vi "Pin Positions DAO.vi"(0 "LBCB Settings Actions":T4, 3 "Config Ref Number":T3, 5 "LBCB Number":T1, 7 "LBCB Pins In":T2={"Pin Positions"=[[0.0, 0.0, 0.0]], "Row Labels"=[]}, 11 "error in (no error)":errorcluster) -> (8 "LBCB Pins Output":T2, 14 "Config Ref Number out":T3, 15 "error out":errorcluster)   [LabVIEW 2013]
uses:
  Metadata/Persistant DAO Actions.ctl
  <vilib>/Utility/config.llb/Config Data RefNum.ctl
  Metadata/Pin Positions.ctl
  Metadata/LBCB Number.ctl
  <vilib>/Utility/config.llb/NI_LVConfig.lvlib
panel:
  in  "Keys":string[](array[string])=["X1", "X2", "Y1", "Z1", "Z2", "Z3"]
  # "Fixed"
  # "Platten"
  # "X"
  # "Z"
  # "X"
  # "Z"
  # "Y"
  # "Y"
  # "Fixed"
  # "Platten"
  # "X"
  # "Z"
  # "X"
  # "Z"
  # "Y"
  # "Y"
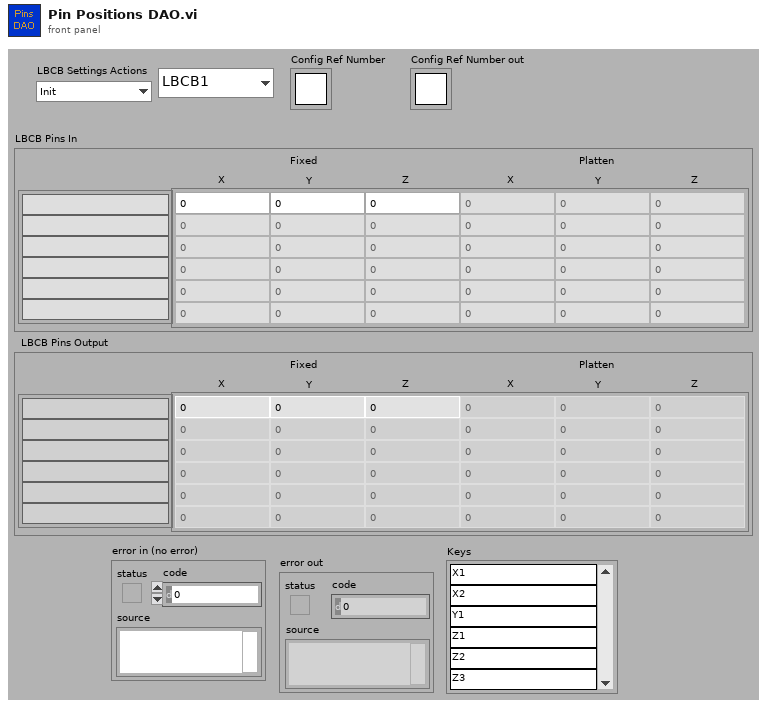
[diagram p1: front panel]
types:
  T1 = typedef "LBCB Number.ctl" = enum16{"LBCB1", "LBCB2"}
  T2 = typedef "Pin Positions.ctl" = cluster{"Pin Positions":dbl[][], "Row Labels":string[]}
  T3 = typedef "NI_LVConfig.lvlib/Config Data RefNum.ctl" = refnum<k1>
  T4 = typedef "Persistant DAO Actions.ctl" = enum16{"Init", "Get", "Set", "Load", "Save"}
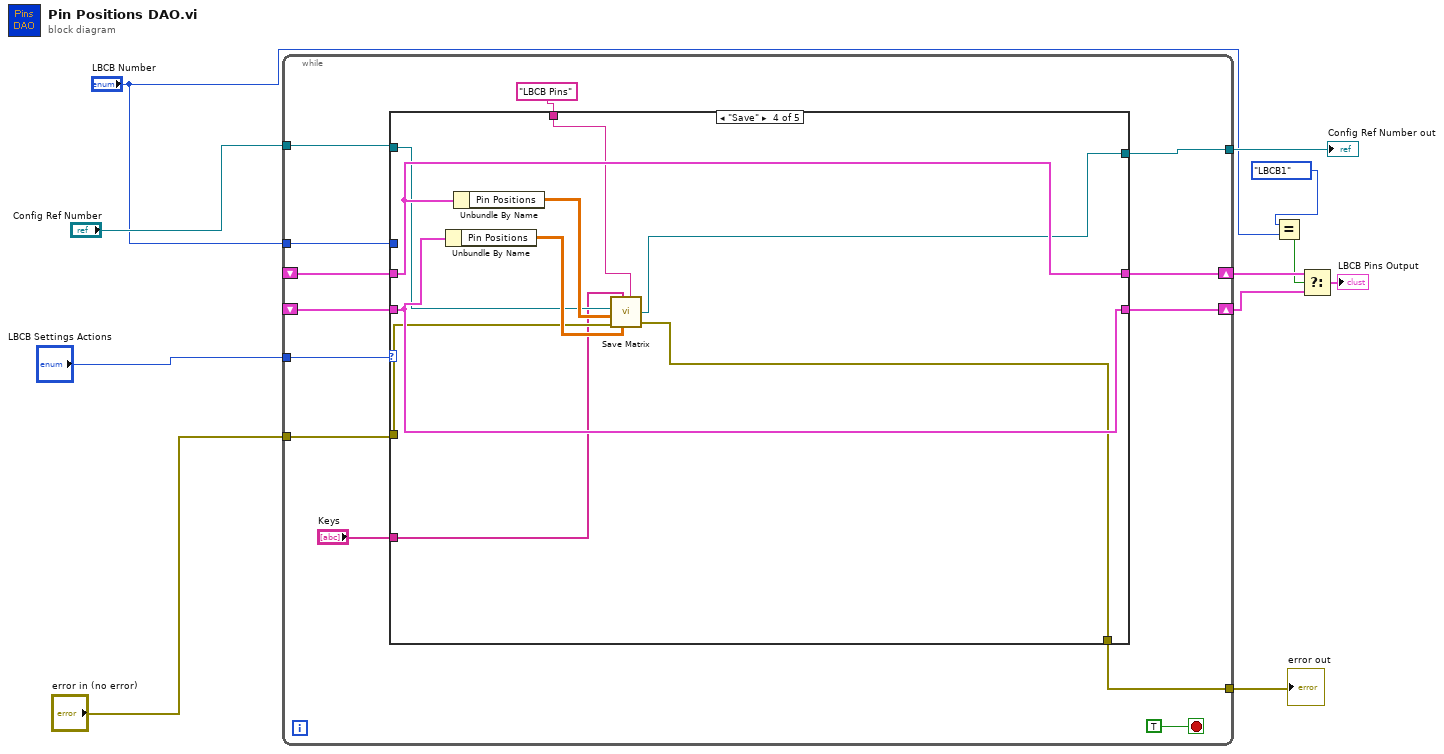
[diagram p0: block diagram]
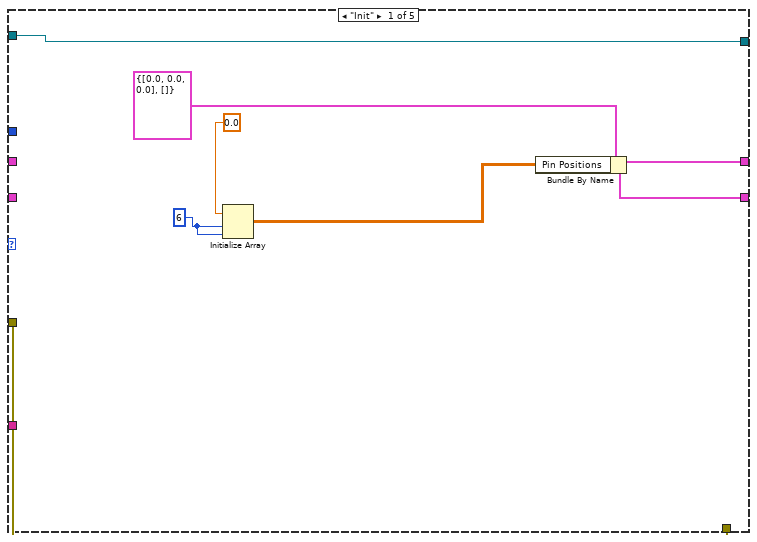
[diagram p2: hidden frame]
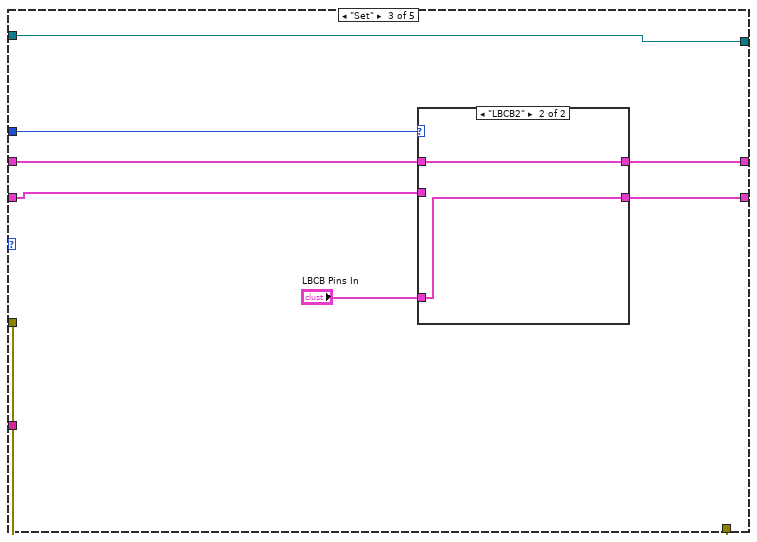
[diagram p4: hidden frame]
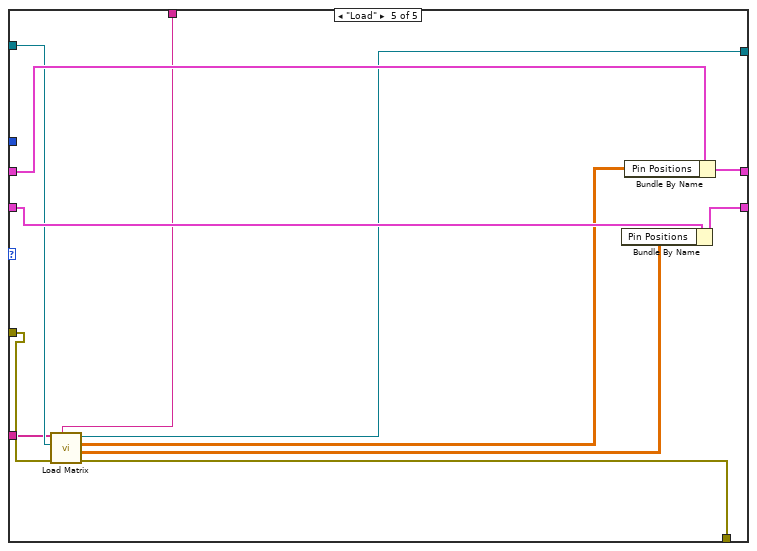
[diagram p6: hidden frame]
diagram:
  n1 = while {
    tunnel: "LBCB Settings Actions" -> [w23]
    tunnel: "Config Ref Number" -> [w22]
    tunnel: "error in (no error)" -> [w20]
    tunnel: [w19] -> w8
    tunnel: [w18] -> w7
    shift-right: [w17] -> w5
    shift-left: _ -> [w16]
    shift-right: [w15] -> w4
    shift-left: _ -> [w14]
    tunnel: "LBCB Number" -> [w13]
    stop <- TRUE stop-if-true
    n2 = case shown="\"Save\"" w23 {
      tunnel: "LBCB Pins" ("section") -> [_ _ _ w50 w64]
      tunnel: w22 -> [w30 w34 w42 w52 w63]
      tunnel: w20 -> [w31 w35 w43 w53 w65]
      tunnel: [w30 w34 w42 w49 w58] -> w19
      tunnel: [w31 w35 w43 w48 w59] -> w18
      tunnel: [w28 w33 w36 w57 w68] -> w17
      tunnel: w16 -> [_ w33 w40 w57 w69]
      tunnel: [w28 w32 w37 w56 w67] -> w15
      tunnel: w14 -> [_ w32 w39 w56 w66]
      tunnel: w13 -> [_ _ w41 _ _]
      tunnel: "Keys" -> [_ _ _ w51 w60]
      frame "Init" {
        w26 = 6 ("index")
        n3 = Initialize Array(0.0 ("element"), w26, w26) -> (w25:dbl[][])
        n4 = Bundle By Name(cluster=T2 {"Pin Positions"=[[0.0, 0.0, 0.0]], "Row Labels"=[]} ("LBCB Settings Output"), "Pin Positions"=w25) -> (w28:T2)
      }
      frame "Get" {
      }
      frame "Set" {
        n5 = case shown="\"LBCB2\"" w41 {
          tunnel: w40 -> [_ w47]
          tunnel: w39 -> [w45 _]
          tunnel: "LBCB Pins In" -> [w44 w46]
          tunnel: [w45 w46] -> w37
          tunnel: [w44 w47] -> w36
          frame "LBCB1" {
          }
          frame "LBCB2" {
          }
        }
      }
      frame "Save" {
        n6 = Unbundle By Name(w56) -> ("Pin Positions"=w54:dbl[][])
        n7 = Unbundle By Name(w57) -> ("Pin Positions"=w55:dbl[][])
        n8 = call "Save Matrix.vi"("section"=w50, "Matrix 2"=w54, "error in (no error)"=w53, "Matrix 1"=w55, "Keys"=w51, "refnum in"=w52) -> ("error out"=w48:errorcluster, "refnum out"=w49:T3)  [unwired: 3 out]
      }
      frame "Load" {
        n9 = call "Load Matrix.vi"("section"=w64, "error in (no error) 2"=w65, "refnum in"=w63, "Keys"=w60) -> ("error in (no error)"=w59:errorcluster, "Matrix 2"=w61:dbl[][], "Matrix 1"=w62:dbl[][], "refnum out"=w58:T3)  [unwired: 4 out]
        n10 = Bundle By Name(cluster=w66, "Pin Positions"=w61) -> (w67:T2)
        n11 = Bundle By Name(cluster=w69, "Pin Positions"=w62) -> (w68:T2)
      }
    }
  }
  "error out" <- w7
  "Config Ref Number out" <- w8
  n12 = Equal?(x=LBCB_Number."LBCB1", y="LBCB Number") -> (x = y?=w3:bool)
  n13 = Select(t=w5, s=w3, f=w4) -> (s? t:f=→"LBCB Pins Output":T2)
